vi "isFull.vi"(8 "error in (no error)":errorcluster, 11 "Bucket in":refnum<class "Bucket.lvclass">) -> (0 "error out":errorcluster, 2 "Full?":bool, 3 "Bucket out":refnum<class "Bucket.lvclass">)   [LabVIEW 2017, in "Bucket.lvclass"]
uses:
  <userlib>/836-Library/Data_Structures/Bucket/Bucket.lvclass
  <userlib>/836-Library/Data_Structures/Bucket/Bucket.lvclass/Bucket.ctl
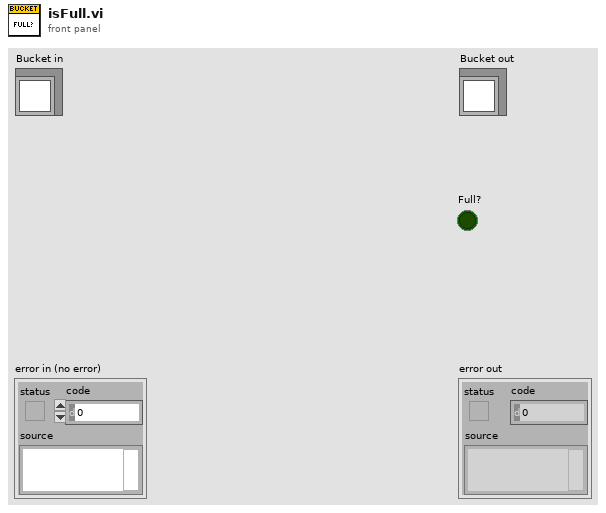
[diagram p1: front panel]
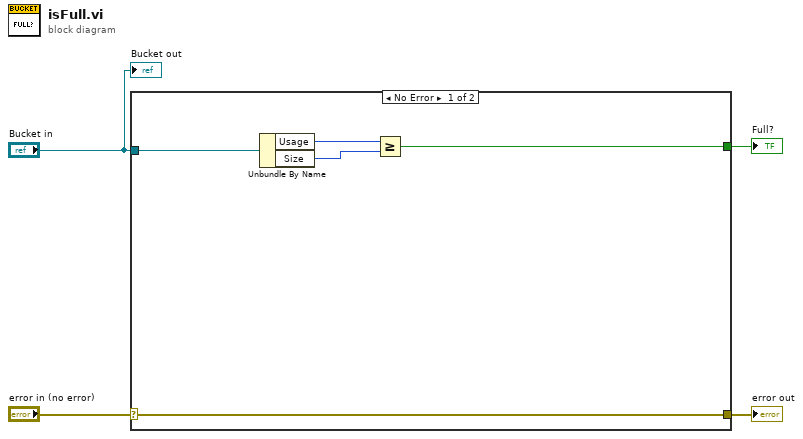
[diagram p0: block diagram]
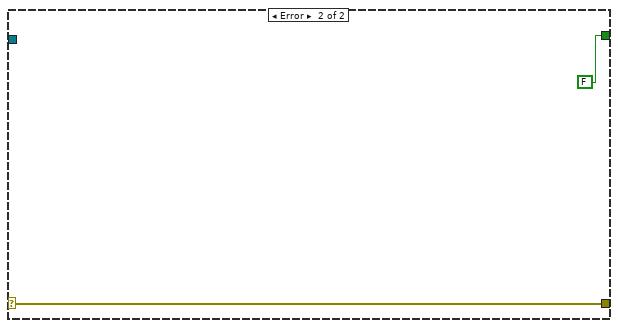
[diagram p2: hidden frame]
diagram:
  n1 = case shown="No Error" "error in (no error)" {
    selector: "error in (no error)" -> [w9 w11]
    tunnel: [w9 w11] -> w3
    tunnel: "Bucket in" -> [w8 _]
    tunnel: [w5 FALSE] -> w2
    frame No Error {
      n2 = Unbundle By Name(w8) -> ("Usage"=w7:u32, "Size"=w6:u32)
      n3 = Greater Or Equal?(x=w7, y=w6) -> (x >= y?=w5:bool)
    }
    frame Error {
    }
  }
  "error out" <- w3
  "Full?" <- w2
  "Bucket out" <- "Bucket in"
